vi "BRig_RT__Case_Exp__State_initTrial__LC_ENL.vi"(6 "input_arrTrig":bool[](array[boolean]), 8 "input_dataTrial":u16[][](array[numeric]), 9 "input_dataExp":u16[](array[numeric]), 10 "input_dataLC":u16[](array[numeric]), 11 "input_dataCurrent":u16[](array[numeric])) -> (0 "output_dataTrial":u16[][](array[numeric]), 3 "output_dataCurrent":u16[](array[numeric]), 4 "output_arrTrig":bool[](array[boolean]))   [LabVIEW 2014]
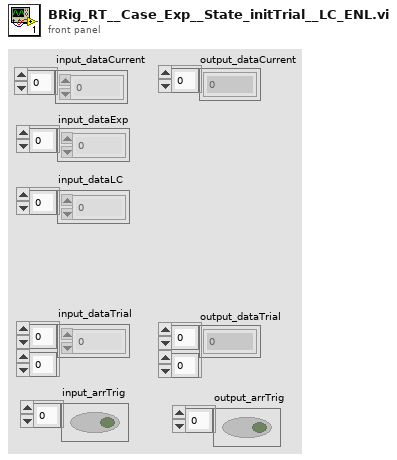
[diagram p1: front panel]
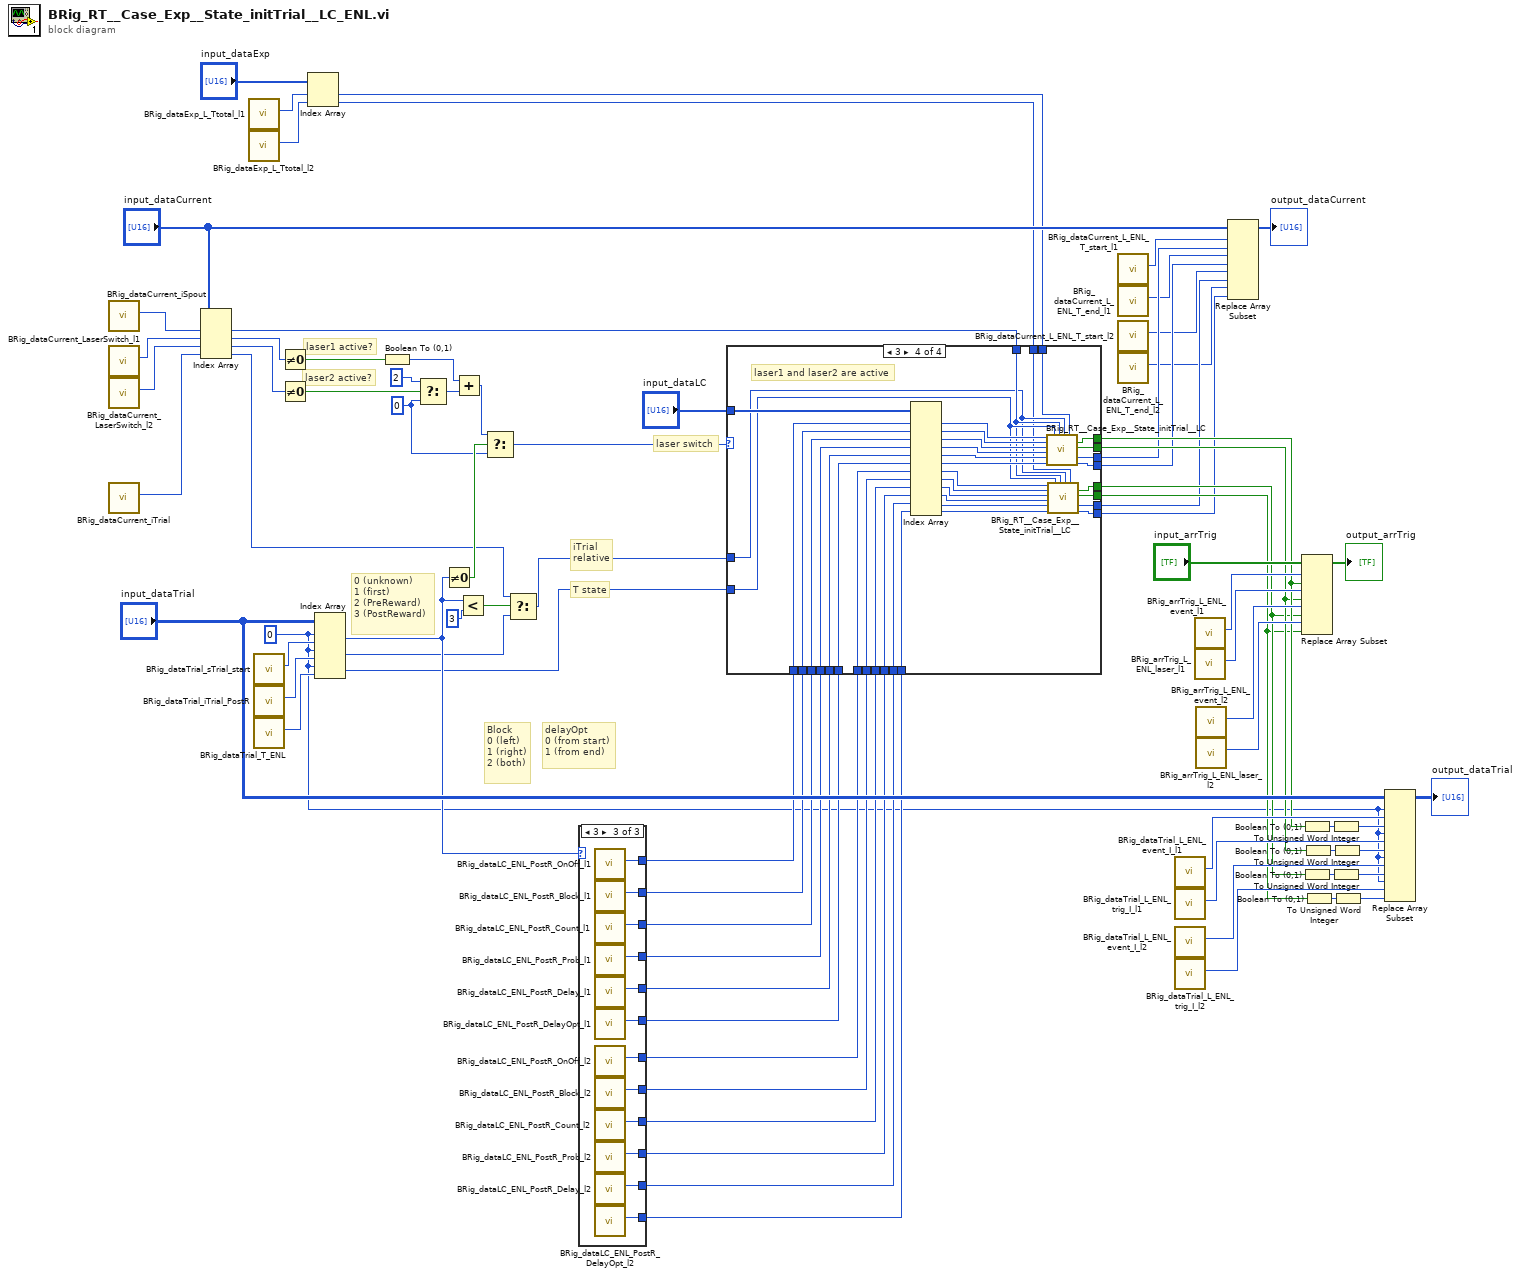
[diagram p0: block diagram]
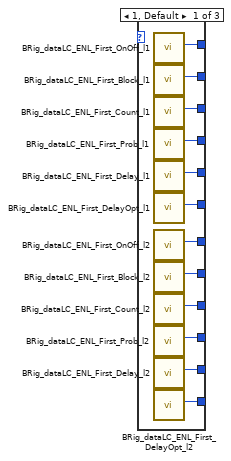
[diagram p2: hidden frame]
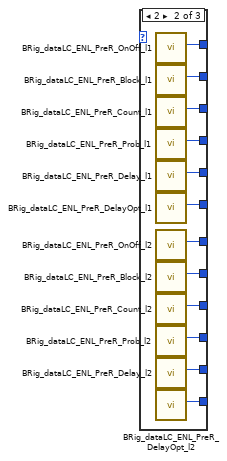
[diagram p3: hidden frame]
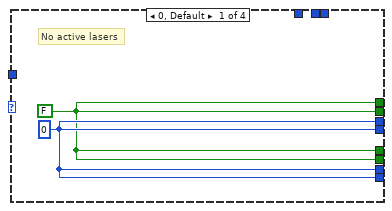
[diagram p4: hidden frame]
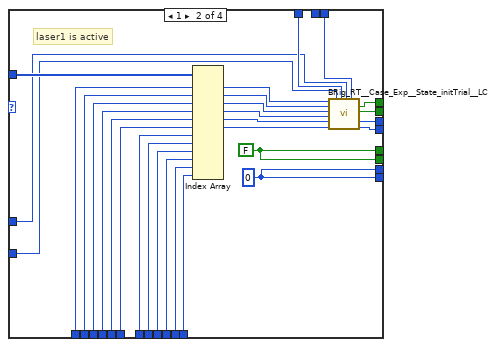
[diagram p5: hidden frame]
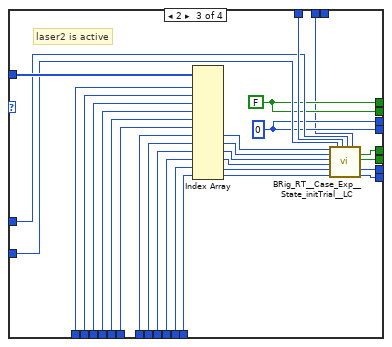
[diagram p6: hidden frame]
diagram:
  w3 = 0
  w68 = i16 0 ("f")
  # "iTrial\nrelative"
  # "laser switch"
  # "T state"
  # "delayOpt\n0 (from start)\n1 (from end)"
  # "Block\n0 (left)\n1 (right)\n2 (both)"
  # "0 (unknown)\n1 (first)\n2 (PreReward)\n3 (PostReward)"
  # "laser2 active?"
  # "laser1 active?"
  n1 = call "BRig_dataCurrent_iSpout.vi"() -> ("output_iSpout"=w64:i32)  [unwired: 11 in]
  n2 = call "BRig_dataCurrent_LaserSwitch_l1.vi"() -> ("output_LaserSwitch_l1"=w79:i32)  [unwired: 11 in]
  n3 = call "BRig_dataCurrent_LaserSwitch_l2.vi"() -> ("output_LaserSwitch_l2"=w78:i32)  [unwired: 11 in]
  n4 = call "BRig_dataCurrent_iTrial.vi"() -> ("output_iTrial"=w2:i32)  [unwired: 11 in]
  n5 = Index Array(array="input_dataCurrent", index #1=w64, index #2=w79, index #3=w78, index #4=w2) -> (element #1=w63:u16, element #2=w77:u16, element #3=w76:u16, element #4=w1:u16)
  n6 = call "BRig_dataExp_L_Ttotal_l1.vi"() -> ("output_L_Ttotal_l1"=w13:i32)  [unwired: 11 in]
  n7 = call "BRig_dataExp_L_Ttotal_l2.vi"() -> ("output_L_Ttotal_l2"=w14:i32)  [unwired: 11 in]
  n8 = call "BRig_dataTrial_sTrial_start.vi"() -> ("output_sTrial_start"=w75:i32)  [unwired: 11 in]
  n9 = call "BRig_dataTrial_iTrial_PostR.vi"() -> ("output_iTrial_PostR"=w7:i32)  [unwired: 11 in]
  n10 = call "BRig_dataTrial_T_ENL.vi"() -> ("output_T_ENL"=w9:i32)  [unwired: 11 in]
  n11 = Not Equal To 0?(x=w77) -> (x != 0?=w74:bool)
  n12 = Not Equal To 0?(x=w76) -> (x != 0?=w73:bool)
  n13 = Index Array(array="input_dataExp", index #1=w13, index #2=w14) -> (element #1=w11:u16, element #2=w10:u16)
  n14 = Index Array(array="input_dataTrial", index (row) #1=w3, index (col) #1=w75, index (row) #2=w3, index (col) #2=w7, index (row) #3=w3, index (col) #3=w9) -> (element #1=w27:u16, element #2=w5:u16, element #3=w8:u16)
  n15 = Boolean To (0,1)(Boolean=w74) -> (0, 1=w70:i16)
  n16 = Select(t=i16 2, s=w73, f=w68) -> (s? t:f=w71:i16)
  n17 = Not Equal To 0?(x=w27) -> (x != 0?=w69:bool)
  n18 = Add(x=w70, y=w71) -> (x+y=w67:i16)
  n19 = Less?(x=w27, y=u16 3) -> (x < y?=w6:bool)
  n20 = Select(t=w67, s=w69, f=w68) -> (s? t:f=w66:i16)
  n21 = Select(t=w1, s=w6, f=w5) -> (s? t:f=w4:u16)
  n22 = case shown="3" w27 {
    tunnel: [w91 w103 w115] -> w26
    tunnel: [w90 w102 w104] -> w25
    tunnel: [w89 w101 w105] -> w24
    tunnel: [w88 w100 w106] -> w23
    tunnel: [w87 w99 w107] -> w22
    tunnel: [w86 w98 w108] -> w21
    tunnel: [w85 w97 w114] -> w20
    tunnel: [w84 w96 w113] -> w19
    tunnel: [w83 w95 w112] -> w18
    tunnel: [w82 w94 w111] -> w17
    tunnel: [w81 w93 w110] -> w16
    tunnel: [w80 w92 w109] -> w15
    frame 1, Default {
      n23 = call "BRig_dataLC_ENL_First_OnOff_l1.vi"() -> ("output_ENL_First_OnOff"=w91:i32)  [unwired: 11 in]
      n24 = call "BRig_dataLC_ENL_First_Block_l1.vi"() -> ("output_ENL_First_Block"=w90:i32)  [unwired: 11 in]
      n25 = call "BRig_dataLC_ENL_First_Count_l1.vi"() -> ("output_ENL_First_Count"=w89:i32)  [unwired: 11 in]
      n26 = call "BRig_dataLC_ENL_First_Prob_l1.vi"() -> ("output_ENL_First_Prob"=w88:i32)  [unwired: 11 in]
      n27 = call "BRig_dataLC_ENL_First_Delay_l1.vi"() -> ("output_ENL_First_Delay"=w87:i32)  [unwired: 11 in]
      n28 = call "BRig_dataLC_ENL_First_DelayOpt_l1.vi"() -> ("output_ENL_First_DelayOpt"=w86:i32)  [unwired: 11 in]
      n29 = call "BRig_dataLC_ENL_First_OnOff_l2.vi"() -> ("output_ENL_First_OnOff_l2"=w85:i32)  [unwired: 11 in]
      n30 = call "BRig_dataLC_ENL_First_Block_l2.vi"() -> ("output_ENL_First_Block_l2"=w84:i32)  [unwired: 11 in]
      n31 = call "BRig_dataLC_ENL_First_Count_l2.vi"() -> ("output_ENL_First_Count_l2"=w83:i32)  [unwired: 11 in]
      n32 = call "BRig_dataLC_ENL_First_Prob_l2.vi"() -> ("output_ENL_First_Prob_l2"=w82:i32)  [unwired: 11 in]
      n33 = call "BRig_dataLC_ENL_First_Delay_l2.vi"() -> ("output_ENL_First_Delay_l2"=w81:i32)  [unwired: 11 in]
      n34 = call "BRig_dataLC_ENL_First_DelayOpt_l2.vi"() -> ("output_ENL_First_DelayOpt_l2"=w80:i32)  [unwired: 11 in]
    }
    frame 2 {
      n35 = call "BRig_dataLC_ENL_PreR_OnOff_l1.vi"() -> ("output_ENL_PreR_OnOff"=w103:i32)  [unwired: 11 in]
      n36 = call "BRig_dataLC_ENL_PreR_Block_l1.vi"() -> ("output_ENL_PreR_Block"=w102:i32)  [unwired: 11 in]
      n37 = call "BRig_dataLC_ENL_PreR_Count_l1.vi"() -> ("output_ENL_PreR_Count"=w101:i32)  [unwired: 11 in]
      n38 = call "BRig_dataLC_ENL_PreR_Prob_l1.vi"() -> ("output_ENL_PreR_Prob"=w100:i32)  [unwired: 11 in]
      n39 = call "BRig_dataLC_ENL_PreR_Delay_l1.vi"() -> ("output_ENL_PreR_Delay"=w99:i32)  [unwired: 11 in]
      n40 = call "BRig_dataLC_ENL_PreR_DelayOpt_l1.vi"() -> ("output_ENL_PreR_DelayOpt"=w98:i32)  [unwired: 11 in]
      n41 = call "BRig_dataLC_ENL_PreR_OnOff_l2.vi"() -> ("output_ENL_PreR_OnOff_l2"=w97:i32)  [unwired: 11 in]
      n42 = call "BRig_dataLC_ENL_PreR_Block_l2.vi"() -> ("output_ENL_PreR_Block_l2"=w96:i32)  [unwired: 11 in]
      n43 = call "BRig_dataLC_ENL_PreR_Count_l2.vi"() -> ("output_ENL_PreR_Count_l2"=w95:i32)  [unwired: 11 in]
      n44 = call "BRig_dataLC_ENL_PreR_Prob_l2.vi"() -> ("output_ENL_PreR_Prob_l2"=w94:i32)  [unwired: 11 in]
      n45 = call "BRig_dataLC_ENL_PreR_Delay_l2.vi"() -> ("output_ENL_PreR_Delay_l2"=w93:i32)  [unwired: 11 in]
      n46 = call "BRig_dataLC_ENL_PreR_DelayOpt_l2.vi"() -> ("output_ENL_PreR_DelayOpt_l2"=w92:i32)  [unwired: 11 in]
    }
    frame 3 {
      n47 = call "BRig_dataLC_ENL_PostR_OnOff_l1.vi"() -> ("output_ENL_PostR_OnOff"=w115:i32)  [unwired: 11 in]
      n48 = call "BRig_dataLC_ENL_PostR_Block_l1.vi"() -> ("output_ENL_PostR_Block"=w104:i32)  [unwired: 11 in]
      n49 = call "BRig_dataLC_ENL_PostR_Count_l1.vi"() -> ("output_ENL_PostR_Count"=w105:i32)  [unwired: 11 in]
      n50 = call "BRig_dataLC_ENL_PostR_Prob_l1.vi"() -> ("output_ENL_PostR_Prob"=w106:i32)  [unwired: 11 in]
      n51 = call "BRig_dataLC_ENL_PostR_Delay_l1.vi"() -> ("output_ENL_PostR_Delay"=w107:i32)  [unwired: 11 in]
      n52 = call "BRig_dataLC_ENL_PostR_DelayOpt_l1.vi"() -> ("output_ENL_PostR_DelayOpt"=w108:i32)  [unwired: 11 in]
      n53 = call "BRig_dataLC_ENL_PostR_OnOff_l2.vi"() -> ("output_ENL_PostR_OnOff_l2"=w114:i32)  [unwired: 11 in]
      n54 = call "BRig_dataLC_ENL_PostR_Block_l2.vi"() -> ("output_ENL_PostR_Block_l2"=w113:i32)  [unwired: 11 in]
      n55 = call "BRig_dataLC_ENL_PostR_Count_l2.vi"() -> ("output_ENL_PostR_Count_l2"=w112:i32)  [unwired: 11 in]
      n56 = call "BRig_dataLC_ENL_PostR_Prob_l2.vi"() -> ("output_ENL_PostR_Prob_l2"=w111:i32)  [unwired: 11 in]
      n57 = call "BRig_dataLC_ENL_PostR_Delay_l2.vi"() -> ("output_ENL_PostR_Delay_l2"=w110:i32)  [unwired: 11 in]
      n58 = call "BRig_dataLC_ENL_PostR_DelayOpt_l2.vi"() -> ("output_ENL_PostR_DelayOpt_l2"=w109:i32)  [unwired: 11 in]
    }
  }
  n59 = case shown="3" w66 {
    tunnel: "input_dataLC" -> [_ w146 w175 w213]
    tunnel: w63 -> [_ w138 w167 w199]
    tunnel: w8 -> [_ w139 w168 w200]
    tunnel: w4 -> [_ w137 w166 w198]
    tunnel: [w116 w136 w149 w197] -> w49
    tunnel: [w116 w135 w149 w196] -> w43
    tunnel: [w117 w134 w148 w195] -> w34
    tunnel: [w117 w133 w148 w194] -> w32
    tunnel: [w116 w120 w165 w193] -> w39
    tunnel: [w117 w119 w164 w192] -> w30
    tunnel: [w116 w120 w163 w191] -> w41
    tunnel: [w117 w119 w162 w190] -> w28
    tunnel: w26 -> [_ w132 w161 w189]
    tunnel: w25 -> [_ w131 w160 w188]
    tunnel: w24 -> [_ w130 w159 w187]
    tunnel: w23 -> [_ w129 w158 w186]
    tunnel: w22 -> [_ w128 w157 w185]
    tunnel: w21 -> [_ w127 w156 w184]
    tunnel: w20 -> [_ w126 w155 w183]
    tunnel: w19 -> [_ w125 w154 w182]
    tunnel: w18 -> [_ w124 w153 w181]
    tunnel: w17 -> [_ w123 w152 w180]
    tunnel: w16 -> [_ w122 w151 w179]
    tunnel: w15 -> [_ w121 w150 w178]
    tunnel: w11 -> [_ w118 _ w177]
    tunnel: w10 -> [_ _ w147 w176]
    frame 0, Default {
      w117 = u16 0
      w116 = FALSE
      # "No active lasers"
    }
    frame 1 {
      w119 = u16 0
      w120 = FALSE
      # "laser1 is active"
      n60 = Index Array(array=w146, index #1=w132, index #2=w131, index #3=w130, index #4=w129, index #5=w128, index #6=w127, index #7=w126, index #8=w125, index #9=w124, index #10=w123, index #11=w122, index #12=w121) -> (element #1=w145:u16, element #2=w144:u16, element #3=w143:u16, element #4=w142:u16, element #5=w141:u16, element #6=w140:u16)  [unwired: 6 out]
      n61 = call "BRig_RT__Case_Exp__State_initTrial__LC.vi"("input_L_OnOff"=w145, "input_L_Block"=w144, "input_L_Count"=w143, "input_L_Prob"=w142, "input_L_Tdelay"=w141, "input_L_delayOpt"=w140, "input_T_state"=w139, "input_iSpout"=w138, "input_iTrial_relative"=w137, "input_L_T"=w118) -> ("output_LC_Event"=w136:bool, "output_LC_Laser"=w135:bool, "output_L_Tstart"=w134:u16, "output_L_Tend"=w133:u16)  [unwired: 6 in]
    }
    frame 2 {
      w148 = u16 0
      w149 = FALSE
      # "laser2 is active"
      n62 = Index Array(array=w175, index #1=w161, index #2=w160, index #3=w159, index #4=w158, index #5=w157, index #6=w156, index #7=w155, index #8=w154, index #9=w153, index #10=w152, index #11=w151, index #12=w150) -> (element #7=w169:u16, element #8=w170:u16, element #9=w171:u16, element #10=w172:u16, element #11=w173:u16, element #12=w174:u16)  [unwired: 6 out]
      n63 = call "BRig_RT__Case_Exp__State_initTrial__LC.vi"("input_L_OnOff"=w169, "input_L_Block"=w170, "input_L_Count"=w171, "input_L_Prob"=w172, "input_L_Tdelay"=w173, "input_L_delayOpt"=w174, "input_T_state"=w168, "input_iSpout"=w167, "input_iTrial_relative"=w166, "input_L_T"=w147) -> ("output_LC_Event"=w163:bool, "output_LC_Laser"=w165:bool, "output_L_Tstart"=w164:u16, "output_L_Tend"=w162:u16)  [unwired: 6 in]
    }
    frame 3 {
      # "laser1 and laser2 are active"
      n64 = Index Array(array=w213, index #1=w189, index #2=w188, index #3=w187, index #4=w186, index #5=w185, index #6=w184, index #7=w183, index #8=w182, index #9=w181, index #10=w180, index #11=w179, index #12=w178) -> (element #1=w212:u16, element #2=w211:u16, element #3=w210:u16, element #4=w209:u16, element #5=w208:u16, element #6=w207:u16, element #7=w201:u16, element #8=w202:u16, element #9=w203:u16, element #10=w204:u16, element #11=w205:u16, element #12=w206:u16)
      n65 = call "BRig_RT__Case_Exp__State_initTrial__LC.vi"("input_L_OnOff"=w212, "input_L_Block"=w211, "input_L_Count"=w210, "input_L_Prob"=w209, "input_L_Tdelay"=w208, "input_L_delayOpt"=w207, "input_T_state"=w200, "input_iSpout"=w199, "input_iTrial_relative"=w198, "input_L_T"=w177) -> ("output_LC_Event"=w197:bool, "output_LC_Laser"=w196:bool, "output_L_Tstart"=w195:u16, "output_L_Tend"=w194:u16)  [unwired: 6 in]
      n66 = call "BRig_RT__Case_Exp__State_initTrial__LC.vi"("input_L_OnOff"=w201, "input_L_Block"=w202, "input_L_Count"=w203, "input_L_Prob"=w204, "input_L_Tdelay"=w205, "input_L_delayOpt"=w206, "input_T_state"=w200, "input_iSpout"=w199, "input_iTrial_relative"=w198, "input_L_T"=w176) -> ("output_LC_Event"=w191:bool, "output_LC_Laser"=w193:bool, "output_L_Tstart"=w192:u16, "output_L_Tend"=w190:u16)  [unwired: 6 in]
    }
  }
  n67 = call "BRig_dataCurrent_L_ENL_T_start_l1.vi"() -> ("output_L_ENL_T_start_l1"=w35:i32)  [unwired: 11 in]
  n68 = call "BRig_dataCurrent_L_ENL_T_end_l1.vi"() -> ("output_L_ENL_T_end_l1"=w33:i32)  [unwired: 11 in]
  n69 = call "BRig_dataCurrent_L_ENL_T_start_l2.vi"() -> ("output_laser2_tENL1_start"=w31:i32)  [unwired: 11 in]
  n70 = call "BRig_dataCurrent_L_ENL_T_end_l2.vi"() -> ("output_L_ENL_T_end_l2"=w29:i32)  [unwired: 11 in]
  n71 = call "BRig_dataTrial_L_ENL_event_I_l1.vi"() -> ("output_L_ENL_event_I_l1"=w50:i32)  [unwired: 11 in]
  n72 = call "BRig_dataTrial_L_ENL_trig_I_l1.vi"() -> ("output_L_ENL_trig_I_l1"=w47:i32)  [unwired: 11 in]
  n73 = call "BRig_dataTrial_L_ENL_event_I_l2.vi"() -> ("output_L_ENL_event_I_l2"=w46:i32)  [unwired: 11 in]
  n74 = call "BRig_dataTrial_L_ENL_trig_I_l2.vi"() -> ("output_L_ENL_trig_I_l2"=w45:i32)  [unwired: 11 in]
  n75 = call "BRig_arrTrig_L_ENL_event_l1.vi"() -> ("output_L_ENL_event_l1"=w59:i32)  [unwired: 11 in]
  n76 = call "BRig_arrTrig_L_ENL_laser_l1.vi"() -> ("output_L_ENL_laserTrig_l1"=w58:i32)  [unwired: 11 in]
  n77 = call "BRig_arrTrig_L_ENL_event_l2.vi"() -> ("output_L_ENL_event_l2"=w57:i32)  [unwired: 11 in]
  n78 = call "BRig_arrTrig_L_ENL_laser_l2.vi"() -> ("output_L_ENL_laserTrig_l2"=w56:i32)  [unwired: 11 in]
  n79 = Replace Array Subset(array="input_dataCurrent", new element #1=w34, index #1=w35, new element #2=w32, index #2=w33, new element #3=w30, index #3=w31, new element #4=w28, index #4=w29) -> (→"output_dataCurrent":u16[])
  n80 = Replace Array Subset(array="input_arrTrig", new element #1=w49, index #1=w59, new element #2=w43, index #2=w58, new element #3=w41, index #3=w57, new element #4=w39, index #4=w56) -> (→"output_arrTrig":bool[])
  n81 = Boolean To (0,1)(Boolean=w49) -> (0, 1=w55:i16)
  n82 = Boolean To (0,1)(Boolean=w41) -> (0, 1=w52:i16)
  n83 = Boolean To (0,1)(Boolean=w43) -> (0, 1=w54:i16)
  n84 = Boolean To (0,1)(Boolean=w39) -> (0, 1=w53:i16)
  n85 = To Unsigned Word Integer(number=w55) -> (unsigned 16bit integer=w48:u16)
  n86 = To Unsigned Word Integer(number=w52) -> (unsigned 16bit integer=w42:u16)
  n87 = To Unsigned Word Integer(number=w54) -> (unsigned 16bit integer=w44:u16)
  n88 = To Unsigned Word Integer(number=w53) -> (unsigned 16bit integer=w40:u16)
  n89 = Replace Array Subset(array="input_dataTrial", new element #1=w48, index (row) #1=w3, index (col) #1=w50, new element #2=w44, index (row) #2=w3, index (col) #2=w47, new element #3=w42, index (row) #3=w3, index (col) #3=w46, new element #4=w40, index (row) #4=w3, index (col) #4=w45) -> (→"output_dataTrial":u16[][])
